vi "test_queue.vi"() -> ()   [LabVIEW 2025]
panel:
  out "Control reading":dbl
  in  "Control works":bool
  in  "488 nm LED control":dbl(slide) step=1.0 scale=0.0..100.0 scale format="%#_3g"
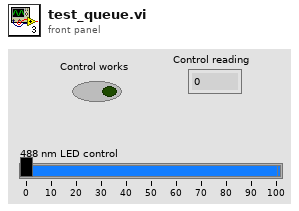
[diagram p1: front panel]
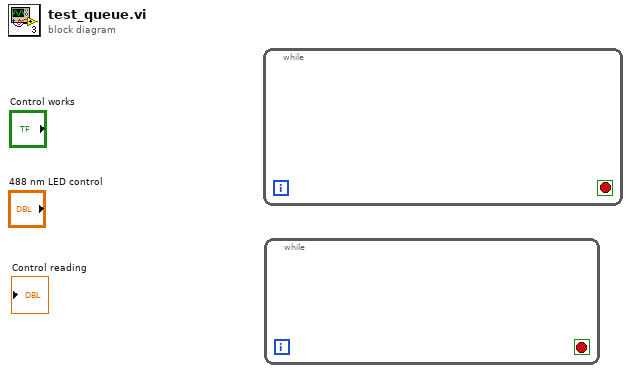
[diagram p0: block diagram]
diagram:
  n1 = while {
    stop <- _ stop-if-true
  }
  n2 = while {
    stop <- _ stop-if-true
  }
